vi "p2.vi"() -> ()   [LabVIEW 2025, in "d12.lvlib"]
uses:
  d12.lvlib
  lv2025-aoc/AOC/AOC.lvlib
panel:
  out "Answer":u64=7670
  in  "Example":string="???.### 1,1,3\n.??..??...?##. 1,1,3\n?#?#?#?#?#?#?#? 1,3,1,6\n????.#...#... 4,1,1\n????.######..#####. 1,6,5\n?###???????? 3,2,1"
  in  "Example":bool
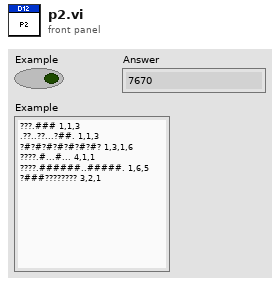
[diagram p1: front panel]
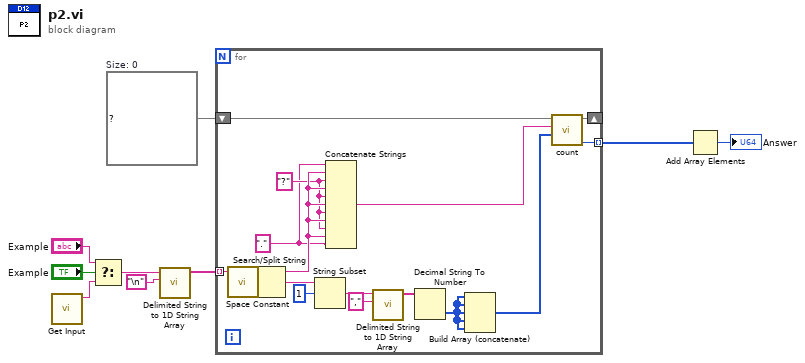
[diagram p0: block diagram]
diagram:
  w1 = map{cluster{string, "nums":i32[]}, u64} {}  # Size: 0
  n1 = call "Get Input.vi"() -> ("Input"=w9:string)  [unwired: 11 in]
  n2 = Select(t="Example", s="Example", f=w9) -> (s? t:f=w8:string)
  n3 = call <vilib>:"Delimited String to 1D String Array.vi"("delimiter"="\n", "delimited string"=w8) -> ("string array"=w4:string[])  [unwired: 9 in]
  n4 = for {
    tunnel: w4 -> [w25] mode=indexing
    tunnel: [w12] -> w2 mode=indexing
    shift-right: [w10] -> _
    shift-left: w1 -> [w11]
    w17 = "." ("string")
    w18 = "?" ("string")
    n5 = call <vilib>:"Space Constant.vi"() -> ("String"=w24:string)
    n6 = Search/Split String(string=w25, search string/char (-)=w24) -> (substring before match=w19:string, match + rest of string=w23:string)  [unwired: 1 in, 1 out]
    n7 = String Subset(string=w23, offset (0)=1) -> (substring=w21:string)  [unwired: 1 in]
    n8 = Concatenate Strings(w17, w19, w18, w19, w18, w19, w18, w19, w18, w19, w17) -> (w14:string)
    n9 = call <vilib>:"Delimited String to 1D String Array.vi"("delimiter"=",", "delimited string"=w21) -> ("string array"=w16:string[])  [unwired: 9 in]
    n10 = Decimal String To Number(string=w16) -> (number=w15:i32[])  [unwired: 2 in, 1 out]
    n11 = Build Array (concatenate)(w15, w15, w15, w15, w15) -> (w13:i32[])
    n12 = call "count.vi"("nums"=w13, "cfg"=w14, "Map in"=w11) -> ("count"=w12:u64, "Map out"=w10:map{cluster{string, "nums":i32[]}, u64})  [unwired: 7 in]
  }
  n13 = Add Array Elements(numeric array=w2) -> (sum=→"Answer":u64)
